vi "Export Error Tree Data.vi"(8 "error in (no error)":errorcluster, 11 "Error Log.lvclass":refnum<class "Error Log.lvclass">) -> (0 "error out":errorcluster, 3 "Error Log.lvclass Out":refnum<class "Error Log.lvclass">)   [LabVIEW 2023, in "Data Analysis.lvlib" / "Error Log.lvlib" / "Error Log.lvclass"]
uses:
  Error Log.lvclass
  Error Log.lvclass/Error Log.ctl
  <userlib>/_OpenG.lib/lvzip/fileutil.llb/subVIs/FILE Delete (Path)__ogtk.vi
  <vilib>/Utility/file.llb/Write Delimited Spreadsheet (string).vi
panel:
  in  "ColHdrs":string[][](array[string])=[["Name", "Error Count"]]
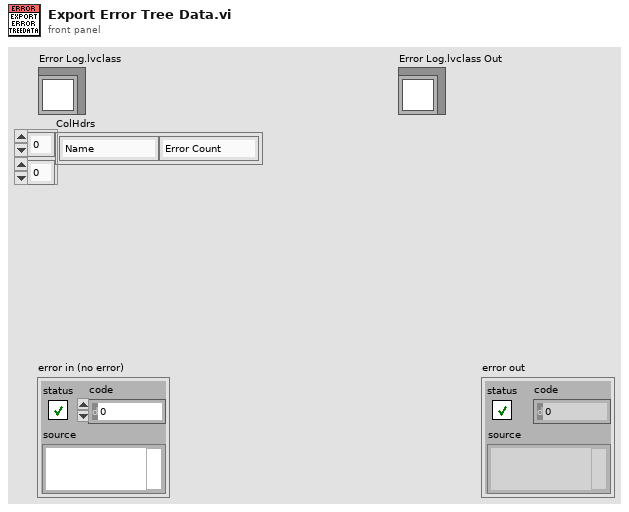
[diagram p1: front panel]
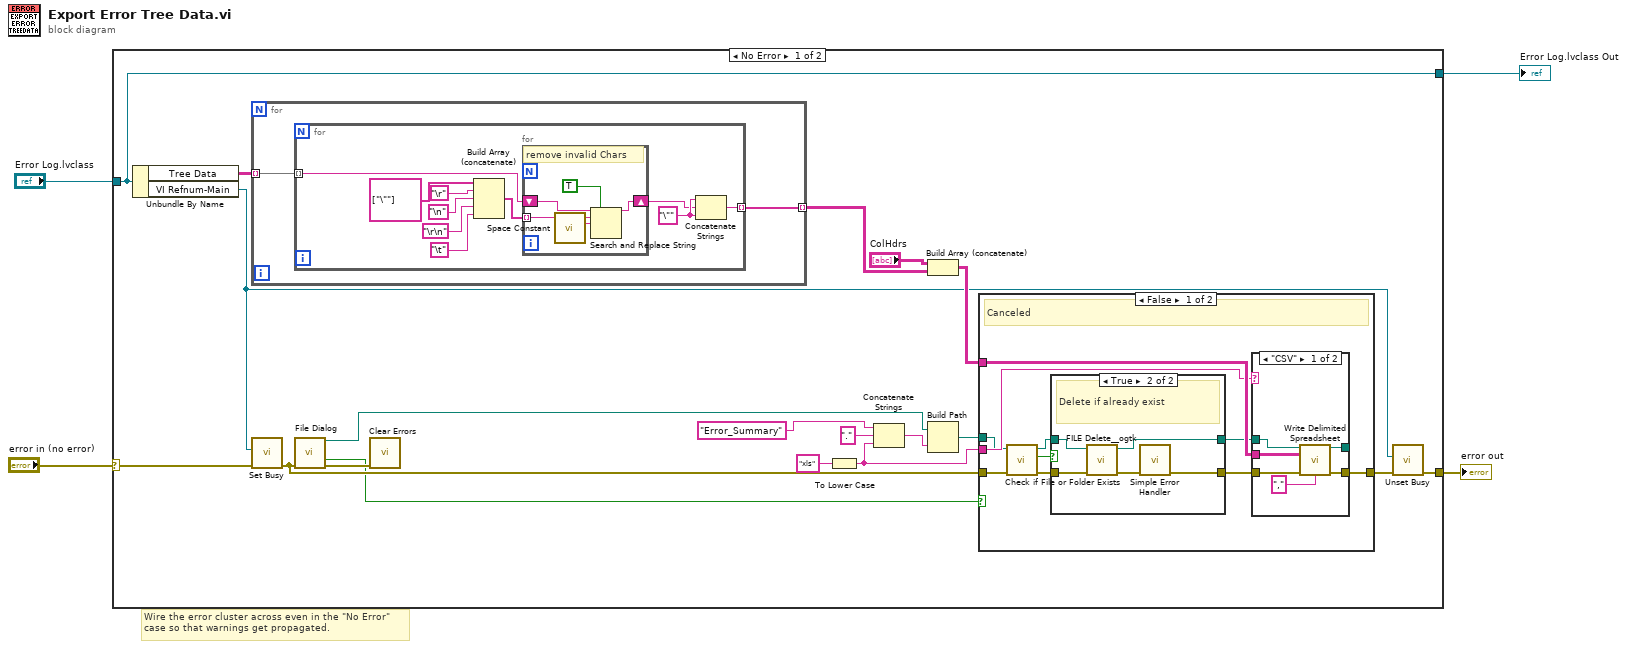
[diagram p0: block diagram]
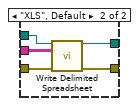
[diagram p3: hidden frame]
diagram:
  # "Wire the error cluster across even in the \"No Error\"\ncase so that warnings get propagated."
  n1 = case shown="No Error" "error in (no error)" {
    selector: "error in (no error)" -> [w22 w71]
    tunnel: [w21 w71] -> w3
    tunnel: [w11 w70] -> w1
    tunnel: "Error Log.lvclass" -> [w11 w70]
    frame No Error {
      n2 = Unbundle By Name(w11) -> ("Tree Data"=w6:string[][], "VI Refnum-Main"=w20:refnum<vi>)
      n3 = for {
        tunnel: w6 -> [w25] mode=indexing
        tunnel: [w24] -> w19 mode=indexing
        n4 = for {
          tunnel: w25 -> [w27] mode=indexing
          tunnel: [w34] -> w24 mode=indexing
          w35 = "\""
          n5 = Build Array (concatenate)(string[] ["\""], "\r", "\n", "\r\n", "\t") -> (w33:string[])
          n6 = for {
            tunnel: w33 -> [w37] mode=indexing
            shift-right: [w38] -> w26
            shift-left: w27 -> [w39]
            # "remove invalid Chars"
            n7 = call <vilib>:"Space Constant.vi"() -> ("String"=w36:string)
            n8 = Search and Replace String(replace all?=TRUE ("replace all? (F)"), input string=w39, search string=w37, replace string=w36) -> (result string=w38:string)  [unwired: 4 in, 3 out]
          }
          n9 = Concatenate Strings(w35, w26, w35) -> (w34:string)
        }
      }
      n10 = call <vilib>:"Set Busy.vi"("error in (no error)"=w22, "VI reference (current VI)"=w20) -> ("error out"=w15:errorcluster)  [unwired: 8 in, 1 out]
      n11 = call "File Dialog"("error in"=w15) -> ("selected path"=w18:path, "cancelled"=w12:bool, "error out"=w14:errorcluster)  [unwired: 11 in, 1 out]
      n12 = call <vilib>:"Clear Errors.vi"("error in (no error)"=w14) -> ()  [unwired: 5 in, 2 out]
      n13 = To Lower Case(string="xls") -> (all lower case string=w7:string)
      n14 = Concatenate Strings("Error_Summary" ("string"), "." ("pattern (all files)"), w7) -> (w16:string)
      n15 = Build Array (concatenate)("ColHdrs", w19) -> (w23:string[][])
      n16 = Build Path(base path=w18, name or relative path=w16) -> (appended path=w13:path)
      n17 = case shown="False" w12 {
        tunnel: w15 -> [w46 w69]
        tunnel: [w50 w69] -> w5
        tunnel: w23 -> [w49 _]
        tunnel: w13 -> [w47 _]
        tunnel: w7 -> [w48 _]
        frame False {
          # "Canceled"
          n18 = call <vilib>:"Check if File or Folder Exists.vi"("error in (no error)"=w46, "path"=w47) -> ("error out"=w44:errorcluster, "file or folder exists?"=w45:bool, "dup path"=w42:path)  [unwired: 7 in]
          n19 = case shown="True" w45 {
            tunnel: w44 -> [w52 w57]
            tunnel: [w52 w53] -> w43
            tunnel: w42 -> [w51 w55]
            tunnel: [w51 w54] -> w41
            frame False {
            }
            frame True {
              # "Delete if already exist"
              n20 = call-poly <userlib>:"FILE Delete__ogtk.vi"("error in (no error)"=w57, "file path"=w55) -> ("error out"=w56:errorcluster, "dup file path"=w54:path)  [unwired: 8 in]
              n21 = call <vilib>:"Simple Error Handler.vi"("error in (no error)"=w56) -> ("error out"=w53:errorcluster)  [unwired: 4 in, 4 out]
            }
          }
          n22 = case shown="\"CSV\"" w48 {
            tunnel: w43 -> [w63 w68]
            tunnel: [w62 w67] -> w50
            tunnel: w49 -> [w59 w66]
            tunnel: w41 -> [w61 w65]
            tunnel: [w58 w64] -> _
            frame "CSV" {
              n23 = call-poly <vilib>:"Write Delimited Spreadsheet.vi"("file path (dialog if empty)"=w61, "2D data"=w59, "error in (no error)"=w63, "delimiter (\\t)"="," ("delimiter (\\t)")) -> ("new file path (Not A Path if cancelled)"=w58:path, "error out"=w62:errorcluster)  [unwired: 10 in]
            }
            frame "XLS", Default {
              n24 = call-poly <vilib>:"Write Delimited Spreadsheet.vi"("file path (dialog if empty)"=w65, "2D data"=w66, "error in (no error)"=w68) -> ("new file path (Not A Path if cancelled)"=w64:path, "error out"=w67:errorcluster)  [unwired: 11 in]
            }
          }
        }
        frame True {
        }
      }
      n25 = call <vilib>:"Unset Busy.vi"("error in (no error)"=w5, "VI reference (current VI)"=w20) -> ("error out"=w21:errorcluster)  [unwired: 9 in]
    }
    frame Error {
    }
  }
  "error out" <- w3
  "Error Log.lvclass Out" <- w1
